vi "Host Image Acquisition Module.vi"(0 "Operation":T3, 11 "error in":errorcluster) -> (1 "Number of Elements to Read Cam Data":u32, 3 "Num Frames read":u32, 4 "Image":T2(plugin-control), 6 "Acq In Progress":bool, 8 "error out":errorcluster, 10 "Image Acquired":bool, 12 "Number of Elements to Write Host DMA":u32, 15 "Frames To Acquire":u32)   [LabVIEW 2013]
uses:
  Host Image Acquisition Module Enum.ctl
  Acquisition Settings Cluster.ctl
  Image Acquisition Settings FG Enum.ctl
  Common/CL Configuration.ctl
  Common/CL Signal Mapping.ctl
  System Status/Status FG Enum.ctl
  Image Processing/Mask ROI FG Enum.ctl
  File IO/Save Image Module Enum.ctl
  Globals/Average Sector Data.vi
  <vilib>/FPGAPlugInAG/PCIe-1473R-LX110/niLvFpga_Reset_PCIe-1473R-LX110.vi
  <vilib>/Utility/error.llb/Error Cluster From Error Code.vi
  <vilib>/rvi/errors/niLvFpgaAdjustHostInterfaceError.vi
  <vilib>/FPGAPlugInAG/PCIe-1473R-LX110/niLvFpga_Run_PCIe-1473R-LX110.vi
  <vilib>/rvi/interface/common/niFpgaWaitOnOcc.vi
  <vilib>/FPGAPlugInAG/PCIe-1473R-LX110/niLvFpga_Close_PCIe-1473R-LX110.vi
  <vilib>/rvi/interface/nirviMethod/nirviMethod.xnode
  FGs/FPGA_Reference.ctl
  FPGA Bitfiles/WBA256Sectors_FPGATarget.lvbitx
  <vilib>/rvi/interface/nirviReadWriteControl/nirviReadWriteControl.xnode
  FPGA/Sector/Accumulate/Sector Parameter Cluster.ctl
  <vilib>/rvi/interface/nirviCloseFPGA/nirviCloseFPGA.xnode
  Common/Timing/Timing Lib.lvlib
  <vilib>/rvi/errors/niLvFpgaMergeErrorWithErrorCode.vi
  NiFpgaLv.dll
  <vilib>/FPGAPlugInAG/PCIe-1473R-LX110/niLvFpga_ReadFifo_PCIe-1473R-LX110.vi
  <vilib>/FPGAPlugInAG/PCIe-1473R-LX110/niLvFpga_ConfigureFifo_PCIe-1473R-LX110.vi
  <vilib>/FPGAPlugInAG/PCIe-1473R-LX110/niLvFpga_StartFifo_PCIe-1473R-LX110.vi
panel:
  out "Actual Depth":u32
  out "Target Sim TO":bool
  out "Cam Data Timeout":bool
  out "Sector FIFO Timeout":bool
  out "Elements Remaining":u32
  out "Words per image":u32
  out "DMA Words per Image":u32
  out "Acquire":bool
  in  "Acquisition Settings Cluster":T1={"Image Width"=1200, "Image Height"=788, "Frames To Acquire"=0, "Signal Mapping"=enum."Basler 10-tap", "DMA Buffer Size\n(In Images)"=2000} {"Image Height" max=65535; "Image Width" max=65535 step=40}
  out "Buffer Size":u32
  out "Acq'd Frame Width":u32=2040
  in  "Start Serial Server":bool
  out "Frames Acq'd":u32=1
  out "Acq'd Frame Height":u32=1088
  out "Initialized":bool
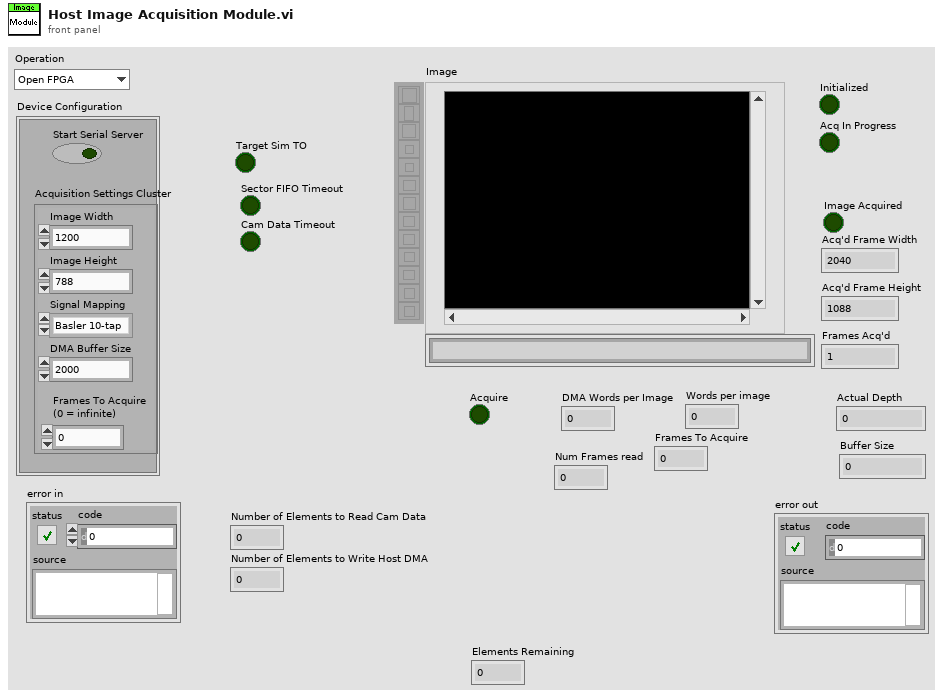
[diagram p1: front panel]
types:
  T1 = typedef "Acquisition Settings Cluster.ctl" = cluster{"Image Width":u32, "Image Height":u32, "Frames To Acquire":u32, "Signal Mapping":enum8{"Standard", "Basler 10-tap", "Vosskühler 10-tap"}, "DMA Buffer Size\n(In Images)":u32}
  T2 = typedef "IMAQ Image.ctl" = refnum<image>
  T3 = typedef "Host Image Acquisition Module Enum.ctl" = enum16{"Open FPGA", "Initialize DMA FIFO", "Load Sim Images", "Initialize Acquisition", "Update Sector Parameters", "Start Acquisition", "Aquire Image", "Read Averages", "Cancel Acquisition", "Close FPGA"}
  T4 = typedef "CL Signal Mapping.ctl" = enum8{"Standard", "Basler 10-tap", "Vosskühler 10-tap"}
  T5 = typedef "CL Configuration.ctl" = enum8{"Base", "Medium", "Full"}
  T6 = typedef "Image Acquisition Settings FG Enum.ctl" = enum16{"Read", "Write"}
  T7 = typedef "Status FG Enum.ctl" = enum16{"Reset", "Read", "Write"}
  T8 = typedef "Mask ROI FG Enum.ctl" = enum16{"Read", "Write", "Enable Background", "Disable Background"}
  T9 = typedef "Save Image Module Enum.ctl" = enum16{"Create File", "Write to File", "Status", "Close File"}
  T10 = typedef "FPGA_Reference.ctl" = refnum<k20>
  T11 = typedef "Mask ROI Cluster.ctl" = cluster{"left annulus":T12, "right annulus":T12, "Threshold Range":cluster{"Lower value":dbl, "Upper value":dbl}, "[Avg BG]":u8[], "Number of Sectors":u8, "Left ROI":T13, "Right ROI":T13, "Left Start Angle Duty Cycle":fxp<+,8,0>, "Left End Angle Duty Cycle":fxp<+,8,0>, "Right End Angle Duty Cycle":fxp<+,8,0>, "Right Start Angle Duty Cycle":fxp<+,8,0>, "[Sector ROIs]":T13[], "Consecutive Sector Threshold":u8}
  T12 = typedef "IMAQ Circle" = cluster{"Center X":i32, "Center Y":i32, "Inner Radius":i32, "Outer Radius":i32, "Start Angle":dbl, "End Angle":dbl}
  T13 = typedef "ROI Descriptor" = cluster{"Global Rectangle":i32[], "Contours":cluster{"ID":enum32{"External", "Internal"}, "Type":u32, "Coordinates":i32[]}[]}
  T14 = typedef "Sector Parameter Cluster.ctl" = cluster{"Start Angle":fxp<+/-,17,2>, "End Angle":fxp<+/-,17,2>, "Inner Radius":u16, "Outter Radius":u16, "Hinge X":u16, "Hinge Y":u16, "NumWingSectors":u8}
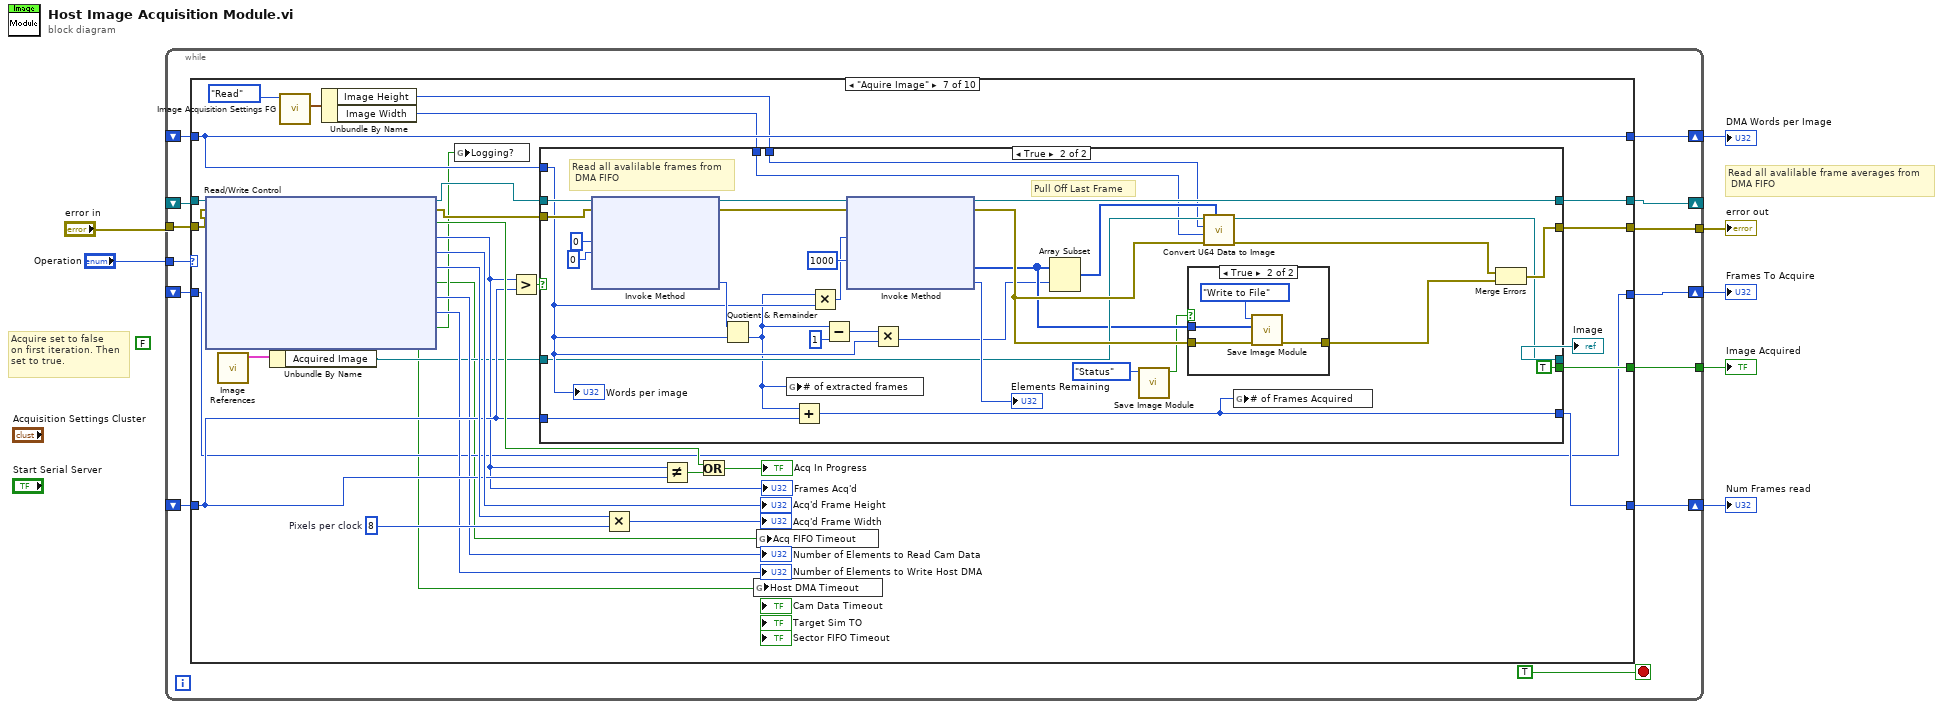
[diagram p0: block diagram]
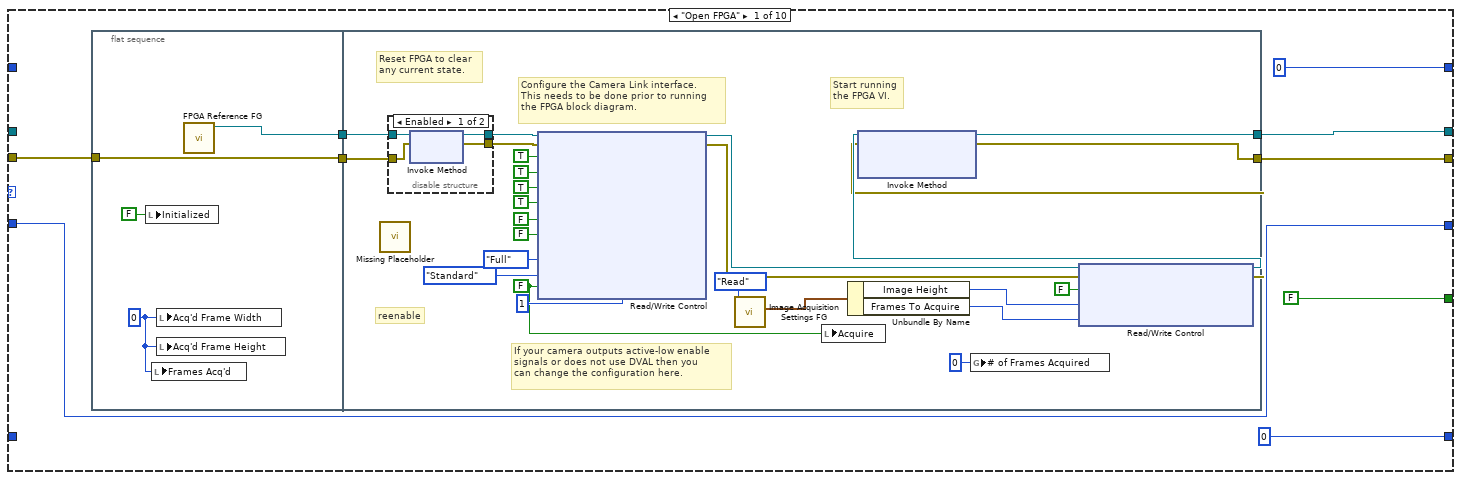
[diagram p2: hidden frame]
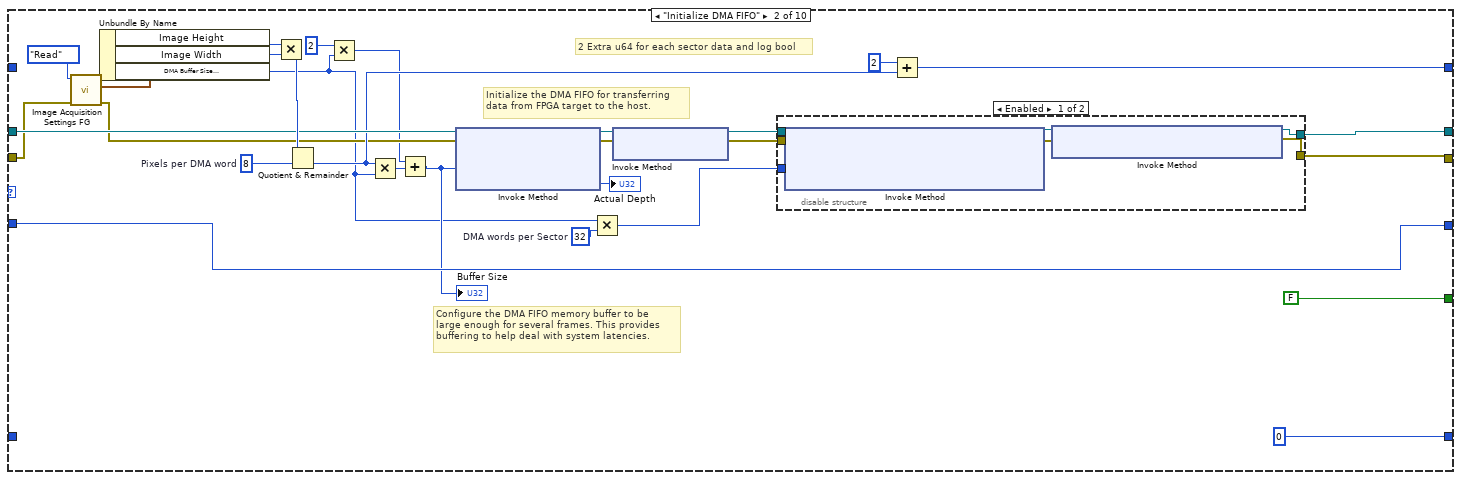
[diagram p4: hidden frame]
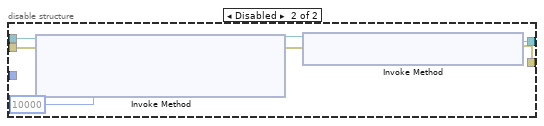
[diagram p5: hidden frame]
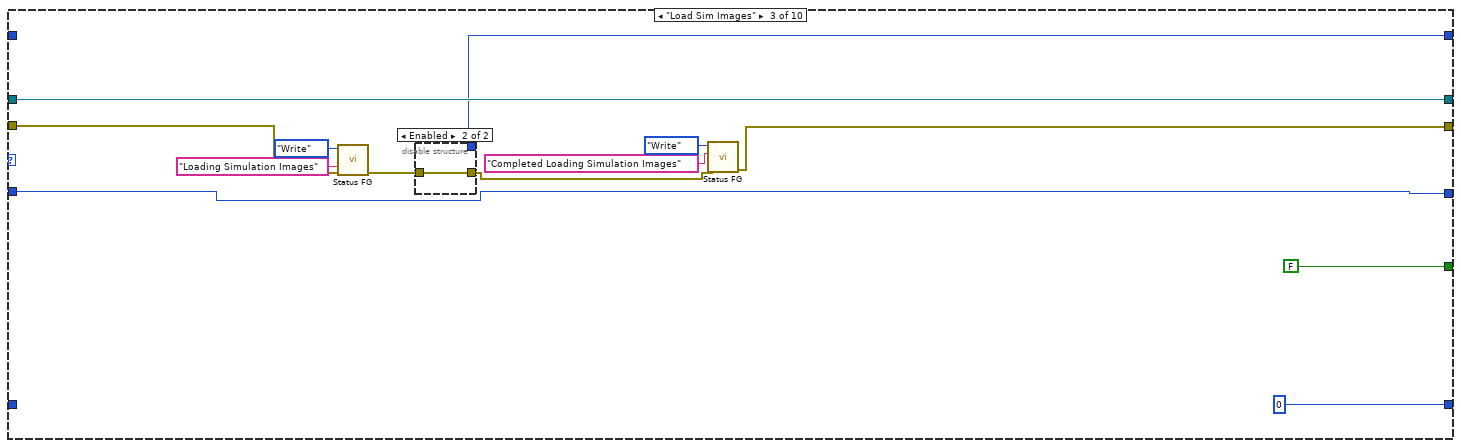
[diagram p6: hidden frame]
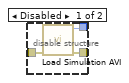
[diagram p7: hidden frame]
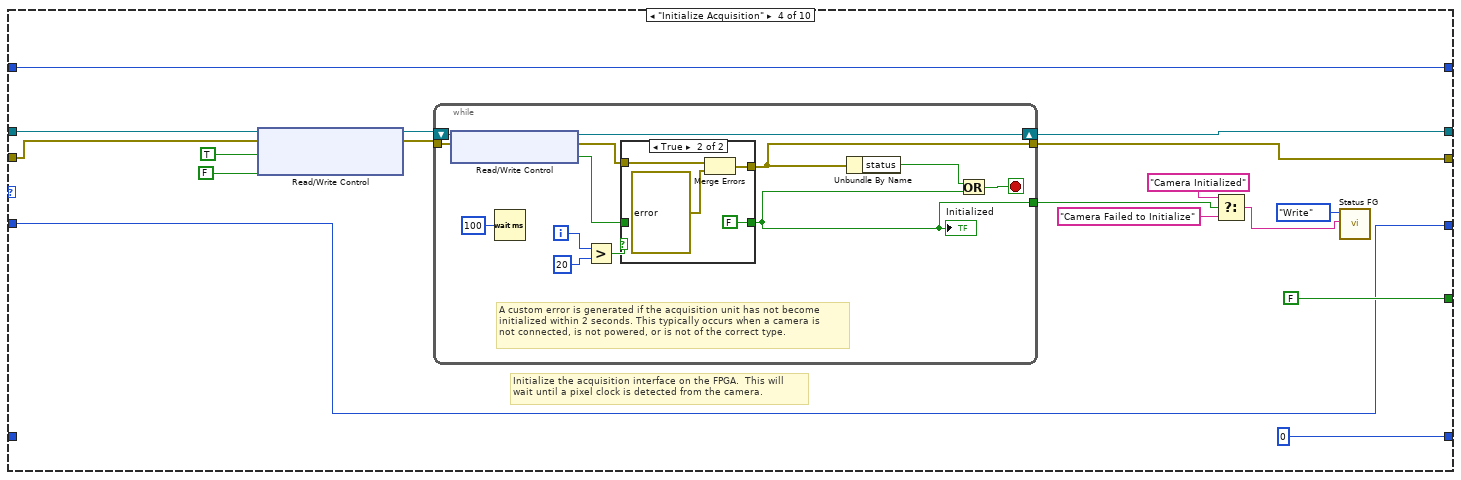
[diagram p8: hidden frame]
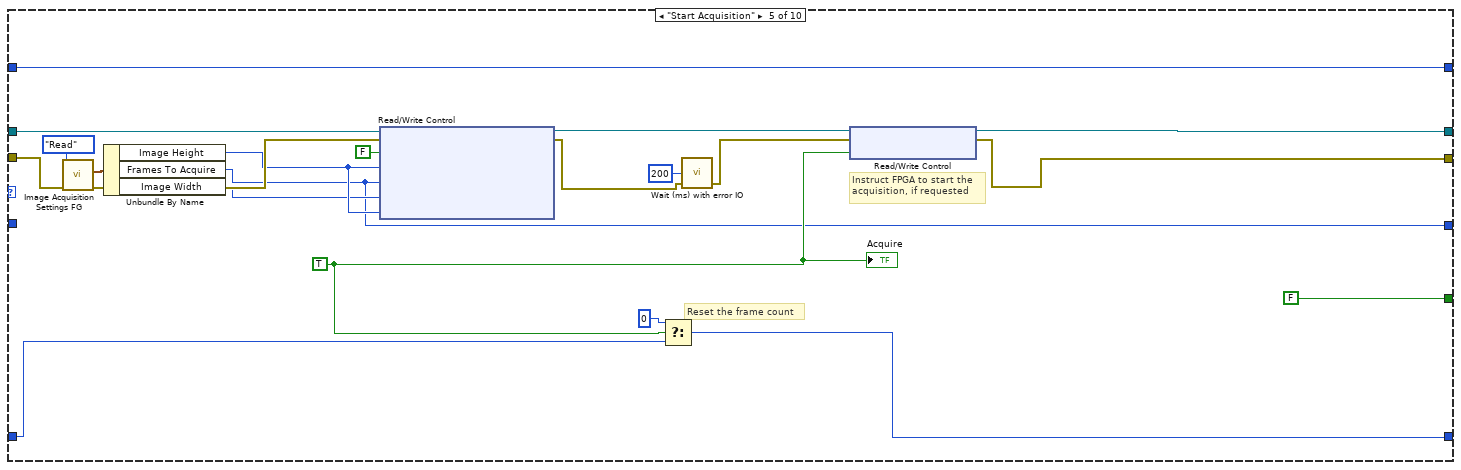
[diagram p10: hidden frame]
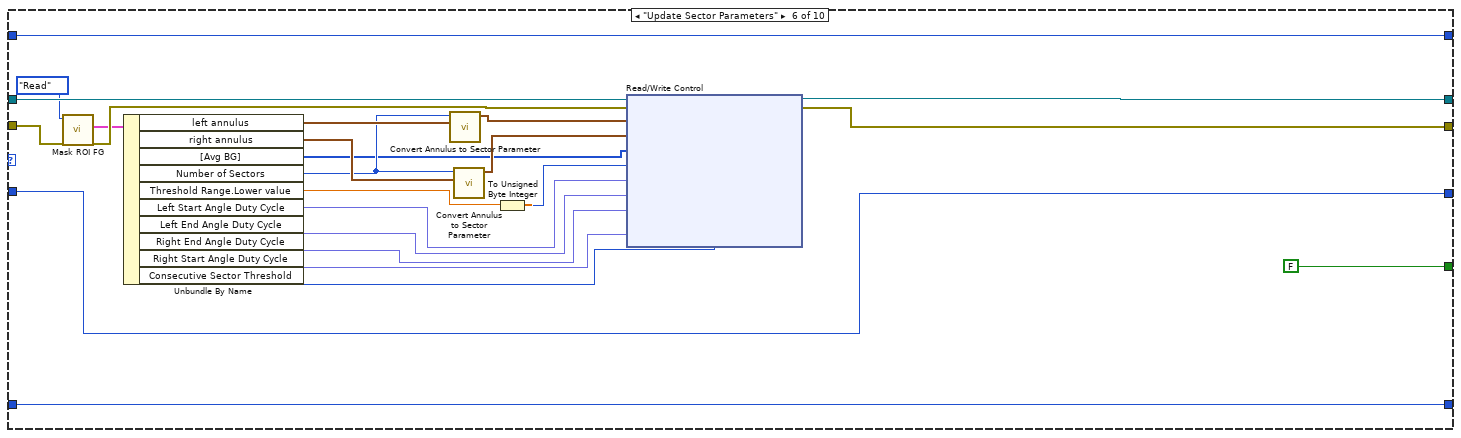
[diagram p11: hidden frame]
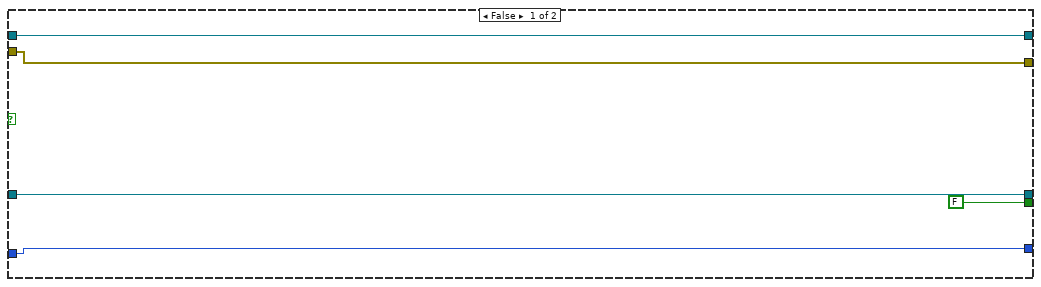
[diagram p12: hidden frame]
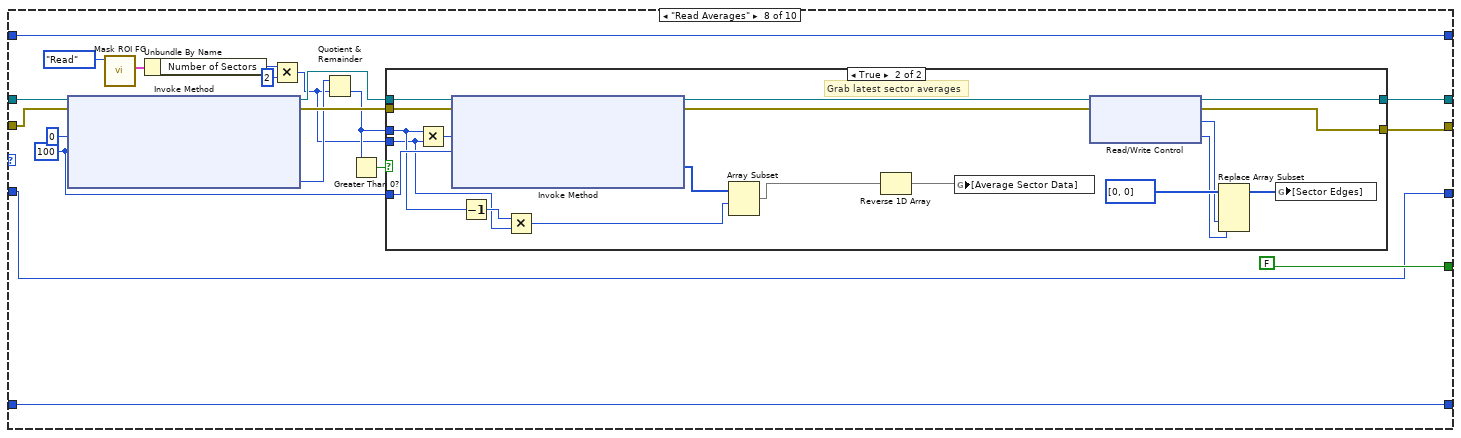
[diagram p14: hidden frame]
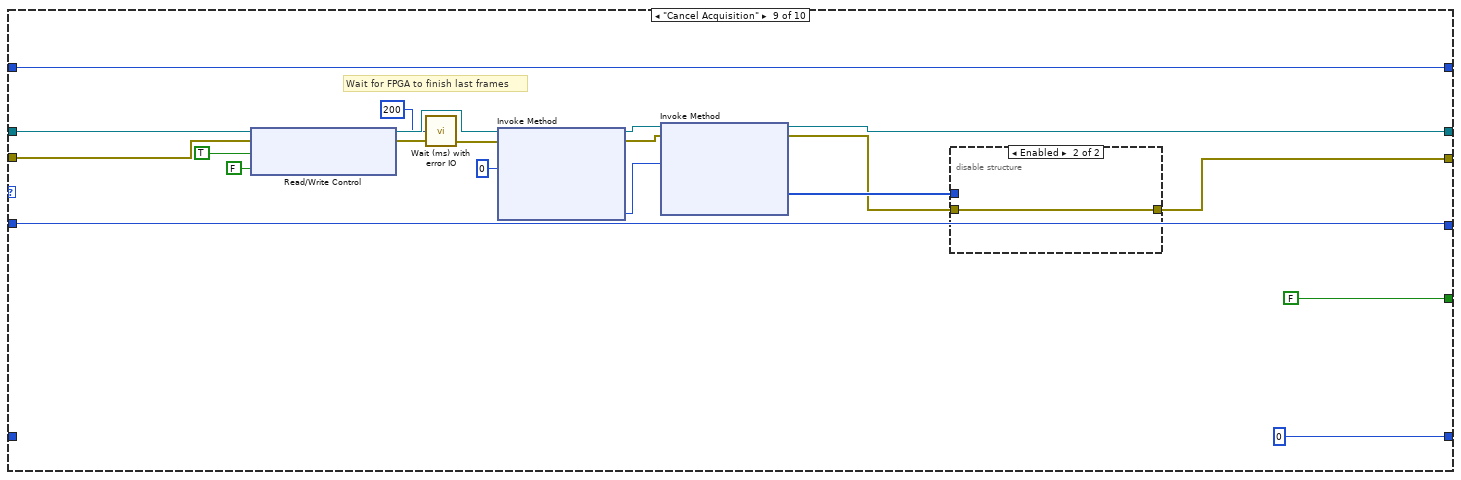
[diagram p16: hidden frame]
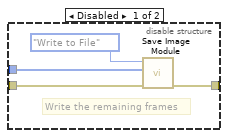
[diagram p17: hidden frame]
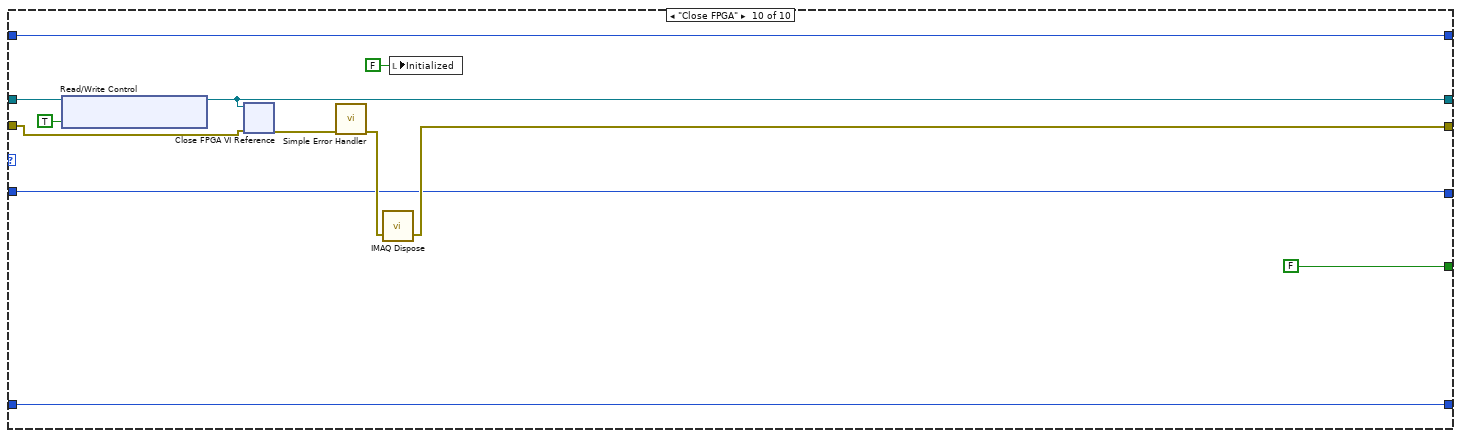
[diagram p18: hidden frame]
diagram:
  (unwired) FALSE ("Acquire")
  # "Read all avalilable frame averages from\n DMA FIFO"
  # "Acquire set to false\non first iteration. Then\nset to true."
  n1 = while {
    shift-right: [w19] -> _
    shift-left: _ -> [w15]
    tunnel: "error in" -> [w18]
    tunnel: "Operation" -> [w17]
    tunnel: [w16] -> w5
    shift-right: [w14] -> w4
    shift-left: _ -> [w13]
    shift-right: [w12] -> w3
    shift-left: _ -> [w11]
    tunnel: [w10] -> w2
    shift-right: [w9] -> w1
    shift-left: _ -> [w8]
    stop <- TRUE stop-if-true
    n2 = case shown="\"Aquire Image\"" w17 {
      tunnel: w18 -> [w29 w85 w117 w133 w177 w204 w223 w293 w338 w348]
      tunnel: [w28 w81 w120 w138 w171 w200 w237 w298 w324 w349] -> w19
      tunnel: [w27 w76 w111 w134 w170 w201 w236 w294 w321 w354] -> w16
      tunnel: w15 -> [_ w90 w120 w139 w178 w206 w238 w299 w340 w351]
      tunnel: [u32 0 w70 w119 w137 w173 w205 w232 w297 w337 w352] -> w14
      tunnel: w13 -> [_ _ _ w137 w173 w205 w232 w297 w337 w352]
      tunnel: [u32 0 u32 0 u32 0 u32 0 w174 w199 w235 w296 u32 0 w353] -> w12
      tunnel: w11 -> [_ _ _ _ w175 w199 w221 w296 _ w353]
      tunnel: [FALSE ("Image Acquired") FALSE ("Image Acquired") FALSE ("Image Acquired") FALSE ("Image Acquired") FALSE ("Image Acquired") FALSE ("Image Acquired") w217 FALSE ("Image Acquired") FALSE ("Image Acquired") FALSE ("Image Acquired")] -> w10
      tunnel: [w21 w73 w109 w126 w162 w184 w211 w292 w333 w346] -> w9
      tunnel: w8 -> [w21 w73 w109 w126 _ w184 w211 w292 w333 w346]
      frame "Open FPGA" {
        n3 = flat-sequence {
          tunnel: w29 -> [w30]
          tunnel: [w31] -> w26
          tunnel: [w30] -> w25
          tunnel: [w48] -> w27
          tunnel: [w49] -> w28
          tunnel: w26 -> [w52]
          tunnel: w25 -> [w50]
          frame #0 {
            w32 = u32 0 ("Acq'd Frame Width")
            n4 = local write "Initialized"(FALSE ("Initialized")) -> ()
            n5 = local write "Frames Acq'd"(w32) -> ()
            n6 = local write "Acq'd Frame Width"(w32) -> ()
            n7 = local write "Acq'd Frame Height"(w32) -> ()
            n8 = call "FPGA Reference FG.vi"() -> ("FPGA VI Reference Out"=w31:T10)  [unwired: 11 in]
          }
          frame #1 {
            w46 = FALSE ("Acq Control.Acquire")
            # "reenable"
            # "If your camera outputs active-low enable\nsignals or does not use DVAL then you \ncan change the configuration here."
            # "Start running\nthe FPGA VI."
            # "Reset FPGA to clear\nany current state."
            # "Configure the Camera Link interface.\nThis needs to be done prior to running\nthe FPGA block diagram."
            n9 = call "Missing Placeholder.vi"() -> ()  [unwired: 12 in]
            n10 = disable-structure shown="Enabled" {
              disable-tunnel: [w63 w65] -> w54
              disable-tunnel: [w62 w64] -> w53
              disable-tunnel: w52 -> [w61 w65]
              disable-tunnel: w50 -> [w60 w64]
              frame Enabled {
                n11 = xnode "Invoke Method"("FPGA VI Reference In"=w61, "error in"=w60) -> ("FPGA VI Reference Out"=w63:T10, "error out"=w62:errorcluster)
              }
              frame Disabled {
              }
            }
            n12 = xnode "Read/Write Control"("FPGA VI Reference In"=w54, "error in"=w53, "CL Config.FVAL Active High"=TRUE ("IO Module Config.CL FVAL Active High"), "CL Config.LVAL Active High"=TRUE ("IO Module Config.CL LVAL Active High"), "CL Config.DVAL Active High"=TRUE ("IO Module Config.CL DVAL Active High"), "CL Config.Spare Active High"=TRUE ("IO Module Config.CL Spare Active High"), "CL Config.Line Scan"=FALSE, "Acq Control.Ignore DVAL"=FALSE ("CL Config.Line Scan"), "CL Config.Configuration"=CL_Configuration."Full", "CL Config.Signal Mapping"=CL_Signal_Mapping."Standard", "Acq Control.Acquire"=w46, "# of Frames to Average"=u8 1) -> ("FPGA VI Reference Out"=w41:T10, "error out"=w39:errorcluster)
            n13 = call "Image Acquisition Settings FG.vi"("Operation"=Image_Acquisition_Settings_FG_Enum."Read") -> ("Acquisition Settings Out"=w45:T1)  [unwired: 9 in, 1 out]
            n14 = local write "Acquire"(w46) -> ()
            n15 = Unbundle By Name(w45) -> ("Image Height"=w43:u32, "Frames To Acquire"=w37:u32)
            n16 = global write "Average Sector Data.vi" "# of Frames Acquired"(u32 0 ("# of Frames Acquired")) -> ()
            n17 = xnode "Read/Write Control"("FPGA VI Reference In"=w41, "error in"=w39, "Acq Control.Cancel Acq"=FALSE, "Acq Control.Line Scan Height"=w43, "Acq Control.Frames To Acq"=w37) -> ("FPGA VI Reference Out"=w40:T10, "error out"=w38:errorcluster)
            n18 = xnode "Invoke Method"("FPGA VI Reference In"=w40, "error in"=w38) -> ("FPGA VI Reference Out"=w49:T10, "error out"=w48:errorcluster)  [unwired: 1 in]
          }
        }
      }
      frame "Initialize DMA FIFO" {
        w75 = u32 32  # DMA words per Sector
        w92 = u32 8  # Pixels per DMA word
        # "2 Extra u64 for each sector data and log bool"
        # "Configure the DMA FIFO memory buffer to be\nlarge enough for several frames. This provides\nbuffering to help deal with system latencies."
        # "Initialize the DMA FIFO for transferring\ndata from FPGA target to the host."
        n19 = call "Image Acquisition Settings FG.vi"("error in (no error)"=w85, "Operation"=Image_Acquisition_Settings_FG_Enum."Read") -> ("error out"=w82:errorcluster, "Acquisition Settings Out"=w86:T1)  [unwired: 8 in]
        n20 = Unbundle By Name(w86) -> ("Image Height"=w84:u32, "Image Width"=w83:u32, "DMA Buffer Size\n(In Images)"=w69:u32)
        n21 = Multiply(x=w84, y=w83) -> (x*y=w91:u32)
        n22 = Quotient & Remainder(x=w91, y=w92) -> (floor(x/y)=w89:u32)  [unwired: 1 out]
        n23 = Multiply(x=u32 2, y=w69) -> (x*y=w67:u32)
        n24 = Multiply(x=w89, y=w69) -> (x*y=w72:u32)
        n25 = Add(x=w67, y=w72) -> (x+y=w71:u32)
        "Buffer Size" <- w71
        n26 = xnode "Invoke Method"("FPGA VI Reference In"=w90, "error in"=w82, "Requested Depth"=w71) -> ("FPGA VI Reference Out"=w94:T10, "error out"=w93:errorcluster, "Actual Depth"=→"Actual Depth":u32)
        n27 = Multiply(x=w69, y=w75) -> (x*y=w74:u32)
        n28 = xnode "Invoke Method"("FPGA VI Reference In"=w94, "error in"=w93) -> ("FPGA VI Reference Out"=w79:T10, "error out"=w77:errorcluster)
        n29 = disable-structure shown="Enabled" {
          disable-tunnel: w74 -> [w101 _]
          disable-tunnel: [w100 w108] -> w81
          disable-tunnel: w79 -> [w99 w107]
          disable-tunnel: w77 -> [w98 w106]
          disable-tunnel: [w95 w103] -> w76
          frame Enabled {
            n30 = xnode "Invoke Method"("FPGA VI Reference In"=w99, "error in"=w98, "Requested Depth"=w101) -> ("FPGA VI Reference Out"=w97:T10, "error out"=w96:errorcluster)  [unwired: 1 out]
            n31 = xnode "Invoke Method"("FPGA VI Reference In"=w97, "error in"=w96) -> ("FPGA VI Reference Out"=w100:T10, "error out"=w95:errorcluster)
          }
          frame Disabled {
            n32 = xnode "Invoke Method"("FPGA VI Reference In"=w107, "error in"=w106, "Requested Depth"=u32 10000) -> ("FPGA VI Reference Out"=w105:T10, "error out"=w104:errorcluster)  [unwired: 1 out]
            n33 = xnode "Invoke Method"("FPGA VI Reference In"=w105, "error in"=w104) -> ("FPGA VI Reference Out"=w108:T10, "error out"=w103:errorcluster)
          }
        }
        n34 = Add(x=u32 2, y=w89) -> (x+y=w70:u32)
      }
      frame "Load Sim Images" {
        n35 = call "Status FG.vi"("error in (no error)"=w117, "Status In"="Loading Simulation Images", "Operation"=Status_FG_Enum."Write") -> ("error out"=w116:errorcluster)  [unwired: 7 in, 1 out]
        n36 = disable-structure shown="Enabled" {
          disable-tunnel: [w124 _] -> w119
          disable-tunnel: w116 -> [w123 w125]
          disable-tunnel: [w122 w125] -> w112
          frame Disabled {
            n37 = call "Load Simulation AVI.vi"("error in (no error)"=w123) -> ("error out"=w122:errorcluster, "Words per image"=w124:u32)  [unwired: 9 in]
          }
          frame Enabled {
          }
        }
        n38 = call "Status FG.vi"("error in (no error)"=w112, "Status In"="Completed Loading Simulation Images", "Operation"=Status_FG_Enum."Write") -> ("error out"=w111:errorcluster)  [unwired: 7 in, 1 out]
      }
      frame "Initialize Acquisition" {
        # "Initialize the acquisition interface on the FPGA.  This will\nwait until a pixel clock is detected from the camera."
        n39 = xnode "Read/Write Control"("FPGA VI Reference In"=w139, "error in"=w133, "Acq Control.Initialize"=TRUE ("Arm Acquisition"), "Acq Control.Cancel Acq"=FALSE) -> ("FPGA VI Reference Out"=w142:T10, "error out"=w141:errorcluster)
        n40 = while {
          tunnel: w141 -> [w150]
          tunnel: [w152] -> w134
          shift-right: [w149] -> w138
          shift-left: w142 -> [w151]
          tunnel: [w143] -> w129
          i -> [w145]
          stop <- w155 stop-if-true
          # "A custom error is generated if the acquisition unit has not become\ninitialized within 2 seconds. This typically occurs when a camera is\nnot connected, is not powered, or is not of the correct type."
          n41 = xnode "Read/Write Control"("FPGA VI Reference In"=w151, "error in"=w150) -> ("FPGA VI Reference Out"=w149:T10, "error out"=w148:errorcluster, "Acq Status.Initialized"=w147:bool)
          n42 = Wait (ms)(milliseconds to wait=u32 100) -> ()  [unwired: 1 out]
          n43 = Greater?(x=w145, y=20) -> (0:w146:bool)
          n44 = case shown="True" w146 {
            tunnel: [w157 FALSE] -> w143
            tunnel: w147 -> [w157 _]
            tunnel: w148 -> [w156 w159]
            tunnel: [w156 w161] -> w152
            frame False {
            }
            frame True {
              n45 = Merge Errors(w159, errorcluster {"status"=TRUE, "code"=-8999, "source"="Acquisition Initialization: This error typically occurs when a camera is not properly connected, is not powered, or is not of the correct type."} ("error in")) -> (w161:errorcluster)
            }
          }
          "Initialized" <- w143
          n46 = Unbundle By Name(w152) -> ("status"=w154:bool)
          n47 = Or(x=w154, y=w143) -> (x .or. y?=w155:bool)
        }
        n48 = Select(t="Camera Initialized", s=w129, f="Camera Failed to Initialize") -> (s? t:f=w131:string)
        n49 = call "Status FG.vi"("Status In"=w131, "Operation"=Status_FG_Enum."Write") -> ()  [unwired: 8 in, 2 out]
      }
      frame "Start Acquisition" {
        w179 = TRUE ("Acquire")
        # "Reset the frame count"
        # "Instruct FPGA to start the\nacquisition, if requested"
        n50 = call "Image Acquisition Settings FG.vi"("error in (no error)"=w177, "Operation"=Image_Acquisition_Settings_FG_Enum."Read") -> ("error out"=w176:errorcluster, "Acquisition Settings Out"=w182:T1)  [unwired: 8 in]
        n51 = Unbundle By Name(w182) -> ("Image Height"=w164:u32, "Frames To Acquire"=w162:u32, "Image Width"=w163:u32)
        n52 = xnode "Read/Write Control"("FPGA VI Reference In"=w178, "error in"=w176, "Acq Control.Cancel Acq"=FALSE, "Acq Control.Line Scan Height"=w164, "Acq Control.Frames To Acq"=w162, "X Resolution"=w163, "Y Resolution"=w164) -> ("FPGA VI Reference Out"=w168:T10, "error out"=w167:errorcluster)
        n53 = Select(t=u32 0, s=w179, f=w175) -> (s? t:f=w174:u32)
        n54 = call "Wait (ms) with error IO.vi"("error in (no error)"=w167, "milliseconds to wait"=u32 200) -> ("error out"=w166:errorcluster)  [unwired: 3 in]
        n55 = xnode "Read/Write Control"("FPGA VI Reference In"=w168, "error in"=w166, "Acq Control.Acquire"=w179) -> ("FPGA VI Reference Out"=w171:T10, "error out"=w170:errorcluster)
        "Acquire" <- w179
      }
      frame "Update Sector Parameters" {
        n56 = call "Mask ROI FG.vi"("error in (no error)"=w204, "Operation"=Mask_ROI_FG_Enum."Read") -> ("error out"=w203:errorcluster, "Mask ROI Out"=w198:T11)  [unwired: 8 in]
        n57 = Unbundle By Name(w198) -> ("left annulus"=w197:T12, "right annulus"=w195:T12, "[Avg BG]"=w192:u8[], "Number of Sectors"=w194:u8, "Threshold Range.Lower value"=w190:dbl, "Left Start Angle Duty Cycle"=w188:fxp<+,8,0>, "Left End Angle Duty Cycle"=w187:fxp<+,8,0>, "Right End Angle Duty Cycle"=w186:fxp<+,8,0>, "Right Start Angle Duty Cycle"=w185:fxp<+,8,0>, "Consecutive Sector Threshold"=w183:u8)
        n58 = call "Convert Annulus to Sector Parameter.vi"("Annulus"=w197, "NumWingSectors"=w194) -> ("Sector Parameter"=w196:T14)  [unwired: 9 in]
        n59 = call "Convert Annulus to Sector Parameter.vi"("Annulus"=w195, "NumWingSectors"=w194) -> ("Sector Parameter"=w193:T14)  [unwired: 9 in]
        n60 = To Unsigned Byte Integer(number=w190) -> (unsigned 8bit integer=w189:u8)
        n61 = xnode "Read/Write Control"("FPGA VI Reference In"=w206, "error in"=w203, "Sector Parameters Left"=w196, "Sector Parameters Right"=w193, "[Average BG Intensity]"=w192, "Sector Threshold"=w189, "Left Start Angle Duty Cycle"=w188, "Left End Angle Duty Cycle"=w187, "Right End Angle Duty Cycle"=w186, "Right Start Angle Duty Cycle"=w185, "Consecutive Sector Threshold"=w183) -> ("FPGA VI Reference Out"=w200:T10, "error out"=w201:errorcluster)
      }
      frame "Aquire Image" {
        w230 = u32 8  # Pixels per clock
        n62 = xnode "Read/Write Control"("FPGA VI Reference In"=w238, "error in"=w223) -> ("FPGA VI Reference Out"=w234:T10, "error out"=w210:errorcluster, "Acq Status.Acq In Progress"=w222:bool, "Acq Status.Frames Acq'd"=w220:u32, "Acq Status.Lines Per Frame"=→"Acq'd Frame Height":u32, "Acq Status.Clocks Per Line"=w229:u32, "Acq FIFO Timeout"=w207:bool, "Number of Elements to Read Cam Data"=→"Number of Elements to Read Cam Data":u32, "Number of Elements to Write Host DMA"=→"Number of Elements to Write Host DMA":u32, "Logging?"=w209:bool, "Host DMA Timeout"=w208:bool)
        "Frames Acq'd" <- w220
        n63 = call "Image References.vi"() -> ("Images"=w214:cluster{"Acquired Image":T2, "Display Image":T2})  [unwired: 10 in, 1 out]
        n64 = Unbundle By Name(w214) -> ("Acquired Image"=w213:T2)
        n65 = call "Image Acquisition Settings FG.vi"("Operation"=Image_Acquisition_Settings_FG_Enum."Read") -> ("Acquisition Settings Out"=w226:T1)  [unwired: 9 in, 1 out]
        n66 = Unbundle By Name(w226) -> ("Image Height"=w225:u32, "Image Width"=w224:u32)
        n67 = global write "Average Sector Data.vi" "Logging?"(w209) -> ()
        n68 = Greater?(x=w220, y=w221) -> (0:w233:bool)
        n69 = case shown="True" w233 {
          tunnel: w234 -> [w242 w271]
          tunnel: w210 -> [w241 w272]
          tunnel: w225 -> [_ w252]
          tunnel: w224 -> [_ w251]
          tunnel: w213 -> [w243 w256]
          tunnel: [w241 w259] -> w236
          tunnel: [w242 w263] -> w237
          tunnel: w221 -> [w240 w274]
          tunnel: [w240 w261] -> w235
          tunnel: w232 -> [_ w264]
          tunnel: [w243 w255] -> w212
          tunnel: [FALSE ("Image Acquired") TRUE ("Image Acquired")] -> w217
          frame False {
          }
          frame True {
            # "Pull Off Last Frame"
            # "Read all avalilable frames from\n DMA FIFO"
            n70 = xnode "Invoke Method"("FPGA VI Reference In"=w271, "error in"=w272, "Number of Elements"=u32 0, "Timeout (ms)"=0) -> ("FPGA VI Reference Out"=w268:T10, "error out"=w267:errorcluster, "Elements Remaining"=w266:u32)  [unwired: 1 out]
            n71 = Quotient & Remainder(x=w266, y=w264) -> (floor(x/y)=w249:u32)  [unwired: 1 out]
            n72 = global write "Average Sector Data.vi" "# of extracted frames"(w249) -> ()
            n73 = Add(x=w249, y=w274) -> (x+y=w261:u32)
            n74 = Multiply(x=w249, y=w264) -> (x*y=w246:u32)
            n75 = Subtract(x=w249, y=u32 1) -> (x-y=w265:u32)
            n76 = xnode "Invoke Method"("FPGA VI Reference In"=w268, "error in"=w267, "Number of Elements"=w246, "Timeout (ms)"=1000) -> ("FPGA VI Reference Out"=w263:T10, "error out"=w257:errorcluster, "Data"=w250:u64[], "Elements Remaining"=→"Elements Remaining":u32)
            n77 = Multiply(x=w265, y=w264) -> (x*y=w248:u32)
            n78 = Array Subset(array=w250, index=w248) -> (w253:u64[])  [unwired: 1 in]
            n79 = call "Save Image Module.vi"("Mode"=Save_Image_Module_Enum."Status") -> ("File Open?"=w244:bool)  [unwired: 9 in, 1 out]
            n80 = case shown="True" w244 {
              tunnel: [w275 w279] -> w258
              tunnel: w257 -> [w275 w278]
              tunnel: w250 -> [_ w277]
              frame False {
              }
              frame True {
                n81 = call "Save Image Module.vi"("error in"=w278, "Data"=w277, "Mode"=Save_Image_Module_Enum."Write to File") -> ("error out"=w279:errorcluster)  [unwired: 7 in, 1 out]
              }
            }
            n82 = call "Convert U64 Data to Image.vi"("Image Data"=w253, "error in"=w257, "Image Width"=w251, "Image Height"=w252, "Image Destination In"=w256) -> ("error out"=w254:errorcluster, "Image Destination Out"=w255:T2)  [unwired: 5 in]
            n83 = global write "Average Sector Data.vi" "# of Frames Acquired"(w261) -> ()
            n84 = Merge Errors(w254, w258) -> (w259:errorcluster)
            "Words per image" <- w264
          }
        }
        "Image" <- w212
        n85 = Multiply(x=w229, y=w230) -> (x*y=→"Acq'd Frame Width":u32)
        n86 = Not Equal?(x=w220, y=w221) -> (x != y?=w219:bool)
        n87 = Or(x=w222, y=w219) -> (x .or. y?=→"Acq In Progress":bool)
        n88 = global write "Average Sector Data.vi" "Host DMA Timeout"(w208) -> ()
        n89 = global write "Average Sector Data.vi" "Acq FIFO Timeout"(w207) -> ()
      }
      frame "Read Averages" {
        w288 = 100 ("Timeout (ms)")
        n90 = xnode "Invoke Method"("FPGA VI Reference In"=w299, "error in"=w293, "Number of Elements"=u32 0, "Timeout (ms)"=w288) -> ("FPGA VI Reference Out"=w290:T10, "error out"=w289:errorcluster, "Elements Remaining"=w283:u32)  [unwired: 1 out]
        n91 = call "Mask ROI FG.vi"("Operation"=Mask_ROI_FG_Enum."Read") -> ("Mask ROI Out"=w286:T11)  [unwired: 9 in, 1 out]
        n92 = Unbundle By Name(w286) -> ("Number of Sectors"=w285:u8)
        n93 = Multiply(x=w285, y=u8 2) -> (x*y=w280:u8)
        n94 = Quotient & Remainder(x=w283, y=w280) -> (floor(x/y)=w281:u32)  [unwired: 1 out]
        n95 = Greater Than 0?(x=w281) -> (x > 0?=w282:bool)
        n96 = case shown="True" w282 {
          tunnel: w290 -> [w301 w320]
          tunnel: w289 -> [w300 w319]
          tunnel: w288 -> [_ w318]
          tunnel: [w301 w314] -> w298
          tunnel: [w300 w315] -> w294
          tunnel: w281 -> [_ w306]
          tunnel: w280 -> [_ w305]
          frame False {
          }
          frame True {
            # "Grab latest sector averages"
            n97 = Multiply(x=w306, y=w305) -> (x*y=w308:u32)
            n98 = xnode "Invoke Method"("FPGA VI Reference In"=w320, "error in"=w319, "Number of Elements"=w308, "Timeout (ms)"=w318) -> ("FPGA VI Reference Out"=w317:T10, "error out"=w316:errorcluster, "Data"=w304:u8[])  [unwired: 1 out]
            n99 = Decrement(x=w306) -> (x-1=w307:u32)
            n100 = Multiply(x=w307, y=w305) -> (x*y=w303:u32)
            n101 = Array Subset(array=w304, index=w303) -> (w302:u8[])  [unwired: 1 in]
            n102 = Reverse 1D Array(array=w302) -> (reversed array=w313:u8[])
            n103 = global write "Average Sector Data.vi" "[Average Sector Data]"(w313) -> ()
            n104 = xnode "Read/Write Control"("FPGA VI Reference In"=w317, "error in"=w316) -> ("FPGA VI Reference Out"=w314:T10, "error out"=w315:errorcluster, "Right Sector Edge"=w311:u16, "Left Sector Edge"=w310:u16)
            n105 = Replace Array Subset(array=u8[] [0, 0] ("[Sector Edges]"), new element #1=w311, new element #2=w310) -> (w309:u8[])  [unwired: 2 in]
            n106 = global write "Average Sector Data.vi" "[Sector Edges]"(w309) -> ()
          }
        }
      }
      frame "Cancel Acquisition" {
        # "Wait for FPGA to finish last frames"
        n107 = xnode "Read/Write Control"("FPGA VI Reference In"=w340, "error in"=w338, "Acq Control.Cancel Acq"=TRUE, "Acq Control.Acquire"=FALSE) -> ("FPGA VI Reference Out"=w326:T10, "error out"=w328:errorcluster)
        n108 = call "Wait (ms) with error IO.vi"("error in (no error)"=w328, "milliseconds to wait"=u32 200) -> ("error out"=w327:errorcluster)  [unwired: 3 in]
        n109 = xnode "Invoke Method"("FPGA VI Reference In"=w326, "error in"=w327, "Number of Elements"=u32 0) -> ("FPGA VI Reference Out"=w331:T10, "error out"=w330:errorcluster, "Elements Remaining"=w329:u32)  [unwired: 1 in, 1 out]
        n110 = xnode "Invoke Method"("FPGA VI Reference In"=w331, "error in"=w330, "Number of Elements"=w329) -> ("FPGA VI Reference Out"=w324:T10, "error out"=w322:errorcluster, "Data"=w323:u64[])  [unwired: 1 in, 1 out]
        n111 = disable-structure shown="Enabled" {
          disable-tunnel: w323 -> [w344 _]
          disable-tunnel: w322 -> [w343 w345]
          disable-tunnel: [w342 w345] -> w321
          frame Disabled {
            # "Write the remaining frames"
            n112 = call "Save Image Module.vi"("error in"=w343, "Data"=w344, "Mode"=Save_Image_Module_Enum."Write to File") -> ("error out"=w342:errorcluster)  [unwired: 7 in, 1 out]
          }
          frame Enabled {
          }
        }
      }
      frame "Close FPGA" {
        n113 = xnode "Read/Write Control"("FPGA VI Reference In"=w351, "Acq Control.Cancel Acq"=TRUE) -> ("FPGA VI Reference Out"=w349:T10)  [unwired: 1 in, 1 out]
        n114 = xnode "Close FPGA VI Reference"("FPGA VI Reference In"=w349, "error in"=w348) -> ("error out"=w357:errorcluster)
        n115 = call <vilib>:"Simple Error Handler.vi"("error in (no error)"=w357) -> ("error out"=w355:errorcluster)  [unwired: 4 in, 4 out]
        n116 = call "IMAQ Dispose"("error in (no error)"=w355) -> ("error out"=w354:errorcluster)  [unwired: 5 in]
        n117 = local write "Initialized"(FALSE ("Initialized")) -> ()
      }
    }
  }
  "error out" <- w5
  "DMA Words per Image" <- w4
  "Num Frames read" <- w3
  "Image Acquired" <- w2
  "Frames To Acquire" <- w1
